vi "Write CSV File.vi"(8 "error in (no error)":errorcluster, 10 "Data":dbl[](array[numeric]), 11 "Path":path) -> (0 "error out":errorcluster)   [LabVIEW 2018]
uses:
  <vilib>/Utility/file.llb/Write Delimited Spreadsheet (DBL).vi
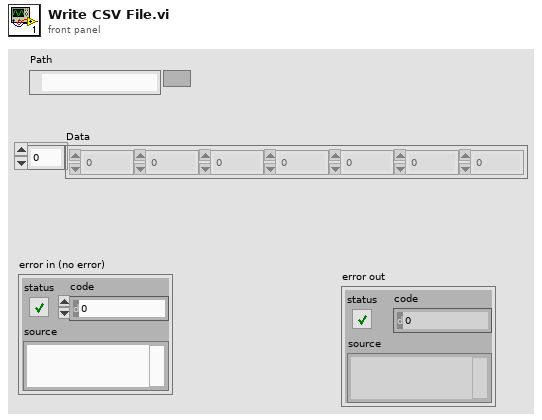
[diagram p1: front panel]
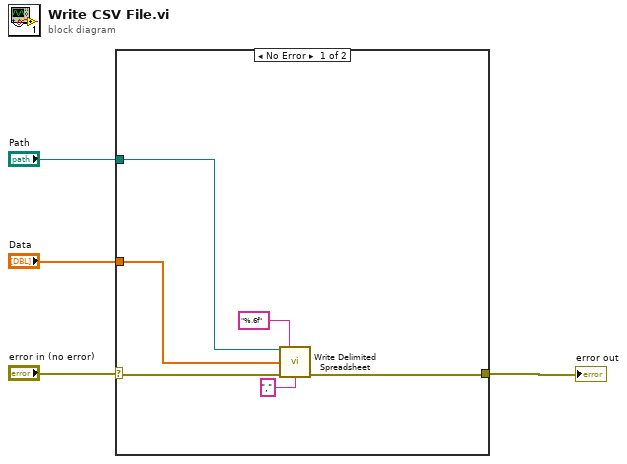
[diagram p0: block diagram]
diagram:
  n1 = case shown="No Error" "error in (no error)" {
    selector: "error in (no error)" -> [w9 w11]
    tunnel: [w10 w11] -> w3
    tunnel: "Path" -> [w8 _]
    tunnel: "Data" -> [w7 _]
    frame No Error {
      n2 = call-poly <vilib>:"Write Delimited Spreadsheet.vi"("file path (dialog if empty)"=w8, "format (%.3f)"="%.6f", "1D data"=w7, "error in (no error)"=w9, "delimiter (\\t)"="," ("delimiter (\\t)")) -> ("error out"=w10:errorcluster)  [unwired: 9 in, 1 out]
    }
    frame Error {
    }
  }
  "error out" <- w3
